vi "Stitching-Generate collage.vi"() -> ()   [LabVIEW 2013]
uses:
  <vilib>/Utility/error.llb/DialogType.ctl
  Coordinates list window/Globals/Coord window-Globals.vi
  Program Files (x86)/National Instruments/LabVIEW 2013/user.lib/My Palettes.lib/Files & paths/Spreadsheet/Read From Spreadsheet File (string)-Mod.vi
panel:
  out "Original data":string[][](array[string])
  # "X"
  # "Y"
  # "X"
  # "Y"
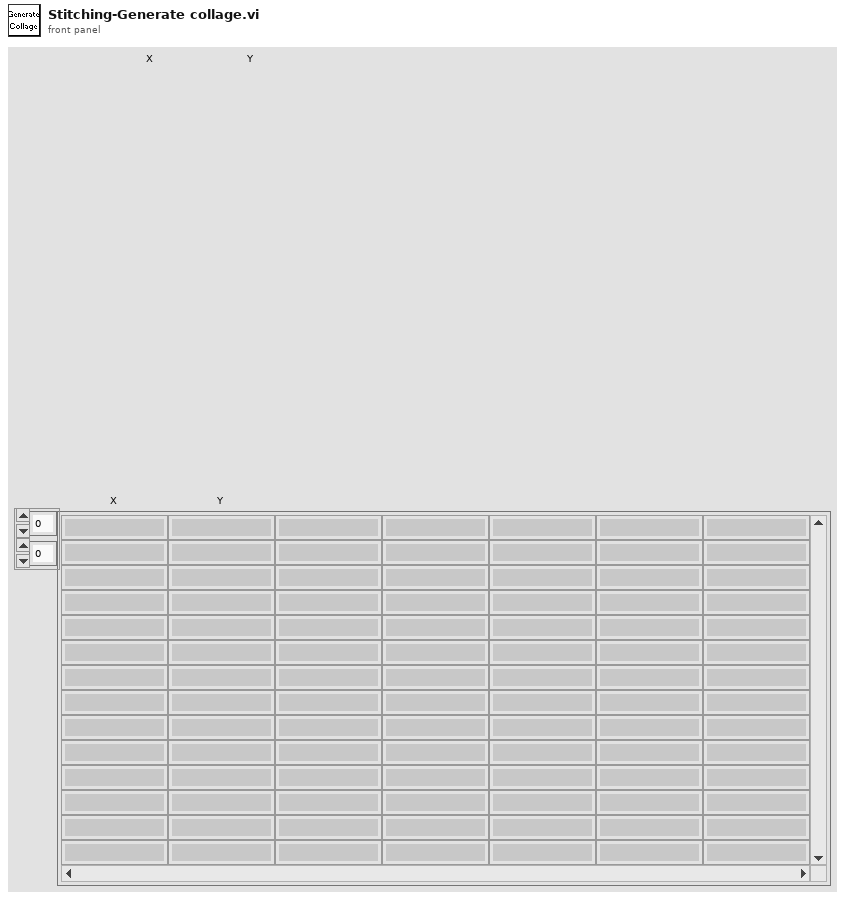
[diagram p1: front panel]
types:
  T1 = typedef "Coordinate list window refs.ctl" = cluster{"Window Name (i.e. Key)":string, "menu reference":refnum<k9>, "VI's reference":refnum<vi>, "Pane 1":refnum<vi>, "Pane 2":refnum<vi>, "Coord Listbox":refnum<vi>, "File name":refnum<vi>, "Picture Map":refnum<vi>, "Stage XYZ Position ind.":refnum<vi>}
  T2 = typedef "Fixed strings.ctl" = cluster{"ROI file name":string, "Normalised ROI file name":string, "Zplane Pockels values file name":string, "Functional data folder name":string, "Experiment Header file name":string, "Z-stack images folder name":string, "Groups setup rel. path":string, "Groups text file rel. path":string, "TDMS files folder name (F.img)":string, "TDMS files folder name (V.acq)":string, "TDMS files folder name (Pl.acq)":string, "Cycle rel times sequence file":string, "Dynamically called VIs folder name":string, "Time Series folder base name":string}
  T3 = typedef "DialogType.ctl" = u16
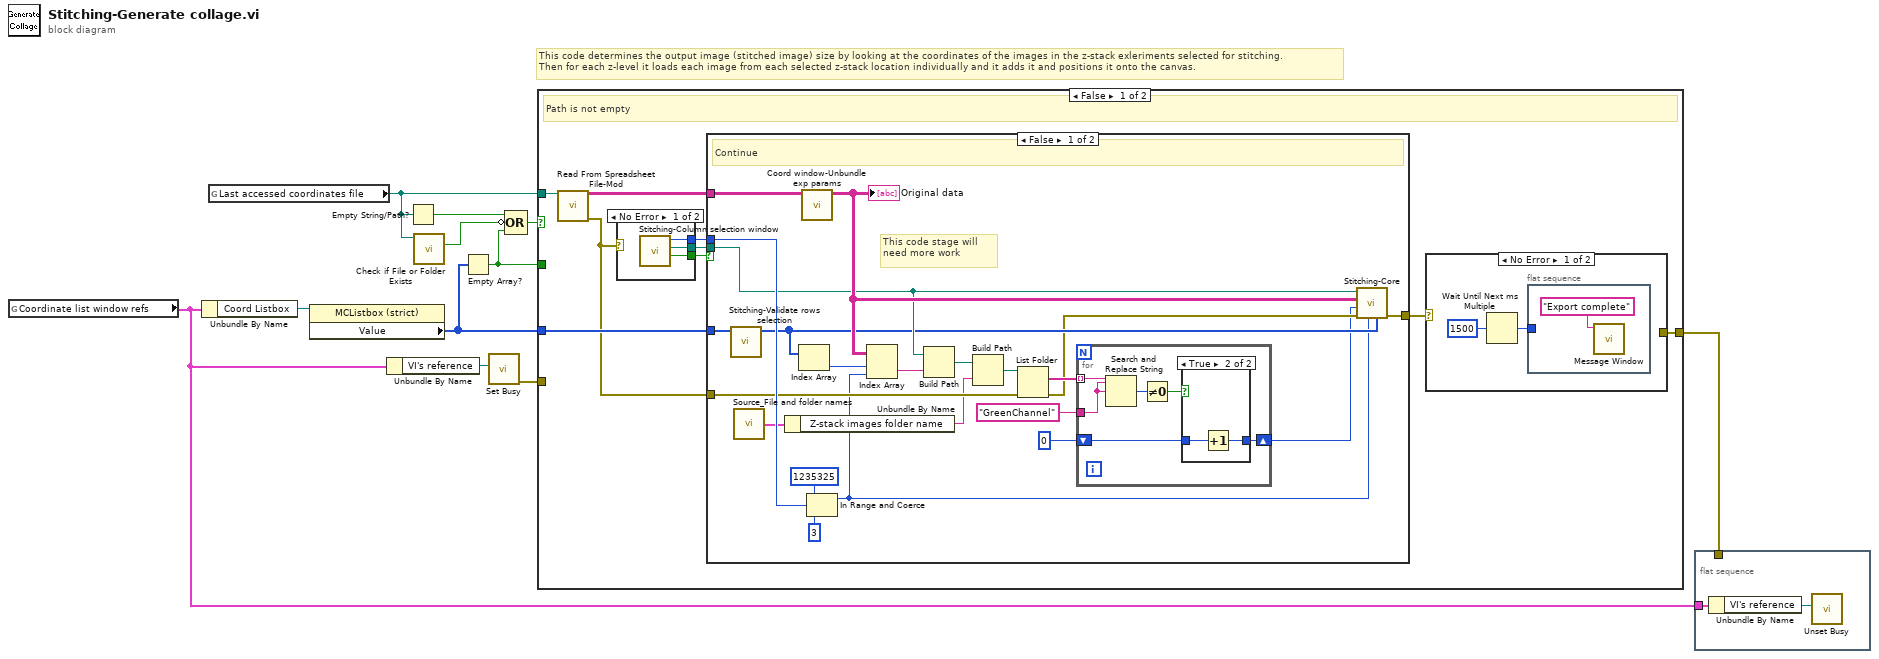
[diagram p0: block diagram]
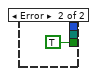
[diagram p4: hidden frame]
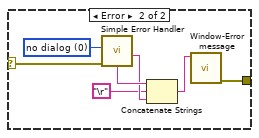
[diagram p5: hidden frame]
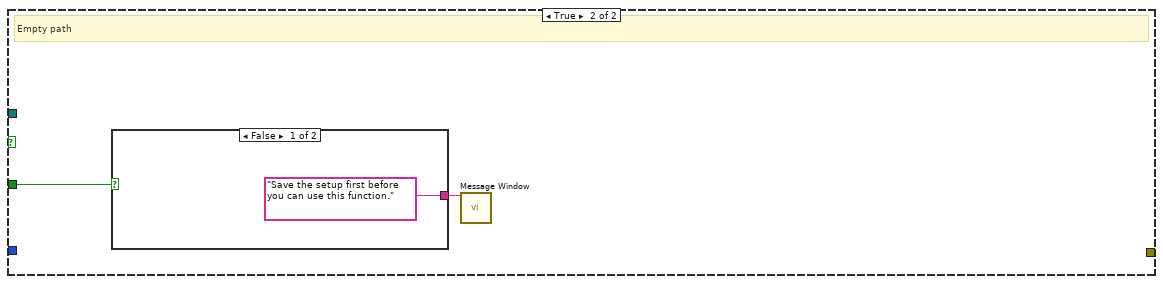
[diagram p6: hidden frame]
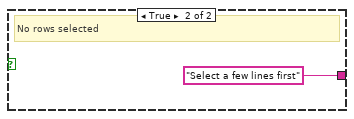
[diagram p7: hidden frame]
diagram:
  # "This code determines the output image (stitched image) size by looking at the coordinates of the images in the z-stack exleriments selected for stitching.\nThen for each z-level it loads each image from each selected z-stack location individually and it adds it and positions it onto the canvas."
  n1 = global read "Coord window-Globals.vi" "Coordinate list window refs"() -> (w3:T1)
  n2 = Unbundle By Name(w3) -> ("Coord Listbox"=w7:refnum<vi>)
  n3 = global read "Coord window-Globals.vi" "Last accessed coordinates file"() -> (w1:path)
  n4 = property class="MCListbox (strict)"(reference=w7) -> ("Value"=w6:i32[])  [unwired: 1 in, 2 out]
  n5 = Unbundle By Name(w3) -> ("VI's reference"=w5:refnum<vi>)
  n6 = Empty String/Path?(string/path=w1) -> (empty?=w10:bool)
  n7 = call <vilib>:"Check if File or Folder Exists.vi"("path"=w1) -> ("file or folder exists?"=w11:bool)  [unwired: 8 in, 2 out]
  n8 = Empty Array?(array=w6) -> (empty?=w8:bool)
  n9 = call <vilib>:"Set Busy.vi"("VI reference (current VI)"=w5) -> ("error out"=w4:errorcluster)  [unwired: 9 in, 1 out]
  n10 = Compound Arithmetic op=OR(w10, invert w11, w8) -> (w9:bool)
  n11 = case shown="False" w9 {
    tunnel: w1 -> [w19 _]
    tunnel: w6 -> [w18 _]
    tunnel: w8 -> [_ w68]
    tunnel: w4 -> [_ _]
    tunnel: [w12 _] -> w2
    frame False {
      # "Path is not empty"
      n12 = call-poly "Read From Spreadsheet File-Mod.vi"("file path (dialog if empty)"=w19) -> ("all rows"=w20:string[][], "error out"=w16:errorcluster)  [unwired: 9 in, 4 out]
      n13 = case shown="No Error" w16 {
        tunnel: [w55 _] -> w15
        tunnel: [w54 TRUE ("Cancelled")] -> w14
        tunnel: [w53 _] -> w13
        frame No Error {
          n14 = call "Stitching-Column selection window.vi"() -> ("Cancelled"=w54:bool, "Base directory"=w53:path, "Column index"=w55:i32)  [unwired: 9 in]
        }
        frame Error {
        }
      }
      n15 = case shown="False" w14 {
        tunnel: w20 -> [w31 _]
        tunnel: w18 -> [w32 _]
        tunnel: [w27 w52] -> w17
        tunnel: w16 -> [w30 w52]
        tunnel: w15 -> [w33 _]
        tunnel: w13 -> [w28 _]
        frame False {
          # "This code stage will need more work"
          # "Continue"
          n16 = call "Stitching-Validate rows selection.vi"("Selected rows indexes in"=w32) -> ("Selected rows indexes"=w26:i32[])  [unwired: 10 in]
          n17 = call "Source_File and folder names.vi"() -> ("Fixed strings"=w22:T2)  [unwired: 1 in]
          n18 = Unbundle By Name(w22) -> ("Z-stack images folder name"=w21:string)
          n19 = Index Array(array=w26) -> (element=w40:i32)  [unwired: 1 in]
          n20 = call "Coord window-Unbundle exp params.vi"("Item Names + exp params"=w31) -> ("Item Names"=w29:string[][])  [unwired: 10 in]
          "Original data" <- w29
          n21 = In Range and Coerce(upper limit=1235325, x=w33, lower limit=3) -> (coerced(x)=w23:i32)  [unwired: 1 out]
          n22 = Index Array(array=w29, index (row)=w40, index (col)=w23) -> (element=w39:string)
          n23 = Build Path(base path=w28, name or relative path=w39) -> (appended path=w38:path)
          n24 = Build Path(base path=w38, name or relative path=w21) -> (appended path=w37:path)
          n25 = List Folder(path=w37, error in=w30) -> (filenames=w36:string[], error out=w25:errorcluster)  [unwired: 2 in, 2 out]
          n26 = for {
            tunnel: w36 -> [w48] mode=indexing
            tunnel: "GreenChannel" ("search string") -> [w47]
            shift-right: [w44] -> w24
            shift-left: 0 -> [w43]
            n27 = Search and Replace String(input string=w48, search string=w47, replace string=w47) -> (number of replacements=w46:i32)  [unwired: 5 in, 3 out]
            n28 = Not Equal To 0?(x=w46) -> (x != 0?=w45:bool)
            n29 = case shown="True" w45 {
              tunnel: [w49 w51] -> w44
              tunnel: w43 -> [w49 w50]
              frame False {
              }
              frame True {
                n30 = Increment(x=w50) -> (x+1=w51:i32)
              }
            }
          }
          n31 = call "Stitching-Core.vi"("selected rows"=w26, "column"=w23, "error in (no error)"=w25, "Z-planes"=w24, "Item Names"=w29, "Base directory containing all dataset folders"=w28) -> ("error out"=w27:errorcluster)  [unwired: 5 in]
        }
        frame True {
          # "Cancelled"
        }
      }
      n32 = case shown="No Error" w17 {
        selector: w17 -> [_ w66]
        tunnel: [_ w64] -> w12
        frame No Error {
          n33 = Wait Until Next ms Multiple(millisecond multiple=u32 1500) -> (millisecond timer value=w58:u32)
          n34 = flat-sequence {
            tunnel: w58 -> [_]
            frame #0 {
              n35 = call "Message Window.vi"("Message string"="Export complete") -> ()  [unwired: 10 in, 1 out]
            }
          }
        }
        frame Error {
          w65 = T3 0 items=["no dialog", "OK message", "continue or stop message", "OK message + warnings", "continue/stop + warnings"] ("type of dialog (OK msg:1)")
          n36 = call <vilib>:"Simple Error Handler.vi"("type of dialog (OK msg:1)"=w65, "error in (no error)"=w66) -> ("source out"=w62:string, "message"=w63:string)  [unwired: 3 in, 3 out]
          n37 = Concatenate Strings(w63, "\r" ("string"), w62) -> (w60:string)
          n38 = call "Window-Error message.vi"("Message"=w60) -> ("Error Out (no error)"=w64:errorcluster)  [unwired: 10 in]
        }
      }
    }
    frame True {
      # "Empty path"
      n39 = case shown="False" w68 {
        tunnel: ["Save the setup first before you can use this function." ("Message string") "Select a few lines first" ("Message string")] -> w67
        frame False {
        }
        frame True {
          # "No rows selected"
        }
      }
      n40 = call "Message Window.vi"("Message string"=w67) -> ()  [unwired: 10 in, 1 out]
    }
  }
  n41 = flat-sequence {
    tunnel: w3 -> [w71]
    tunnel: w2 -> [_]
    frame #0 {
      n42 = Unbundle By Name(w71) -> ("VI's reference"=w72:refnum<vi>)
      n43 = call <vilib>:"Unset Busy.vi"("VI reference (current VI)"=w72) -> ()  [unwired: 10 in, 1 out]
    }
  }
